vi "ParseWeek.vi"(1 "HTML  Body":string) -> (0 "ComicURLs":string[](array[string]))   [LabVIEW 2022 SP3]
uses:
  <vilib>/Utility/error.llb/Trim Whitespace One-Sided.vi
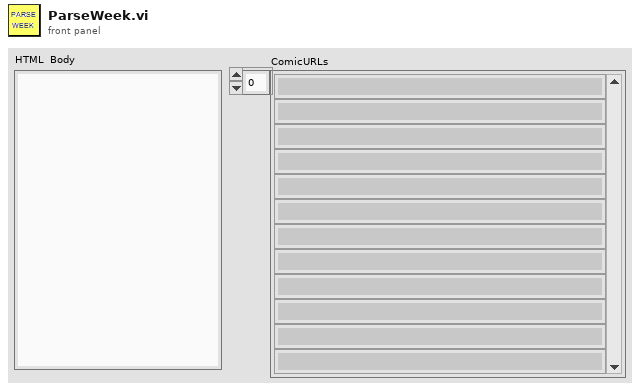
[diagram p1: front panel]
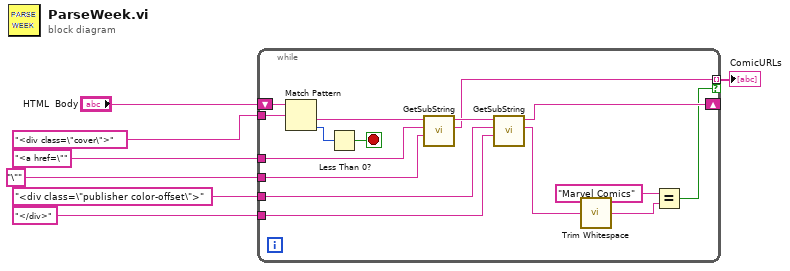
[diagram p0: block diagram]
diagram:
  n1 = while {
    tunnel: "<div class=\"cover\">" -> [w18]
    tunnel: "<a href=\"" -> [w16]
    tunnel: "\"" -> [w10]
    shift-right: [w11] -> _
    shift-left: "HTML  Body" -> [w19]
    tunnel: "<div class=\"publisher color-offset\">" -> [w14]
    tunnel: "</div>" -> [w13]
    tunnel: [w8] -> w1 mode=indexing if=w9
    stop <- w22 stop-if-true
    n2 = Match Pattern(string=w19, regular expression=w18) -> (after substring=w17:string, offset past match=w23:i32)  [unwired: 1 in, 2 out]
    n3 = Less Than 0?(x=w23) -> (x < 0?=w22:bool)
    n4 = call "GetSubString.vi"("End Search"=w10, "Start Search"=w16, "String In"=w17) -> ("Match"=w8:string, "Following String Out"=w15:string)  [unwired: 6 in, 1 out]
    n5 = call "GetSubString.vi"("End Search"=w13, "Start Search"=w14, "String In"=w15) -> ("Match"=w12:string, "Following String Out"=w11:string)  [unwired: 6 in, 1 out]
    n6 = call <vilib>:"Trim Whitespace.vi"("string"=w12) -> ("trimmed string"=w20:string)  [unwired: 1 in]
    n7 = Equal?(x="Marvel Comics", y=w20) -> (x = y?=w9:bool)
  }
  "ComicURLs" <- w1
